vi "plot_read_output_file.vi"(9 "TMP Filepath":path, 10 "Plot Tree":refnum<vi>, 11 "Output File Loaded?":refnum<vi>) -> (3 "# Lines Plot":i32)   [LabVIEW 2019]
uses:
  lib/libOutputReader.so
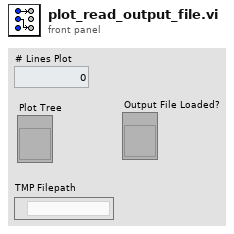
[diagram p1: front panel]
types:
  T1 = cluster{string, string[], "Child Tag":string, i32, "Child Only?":bool, i32}
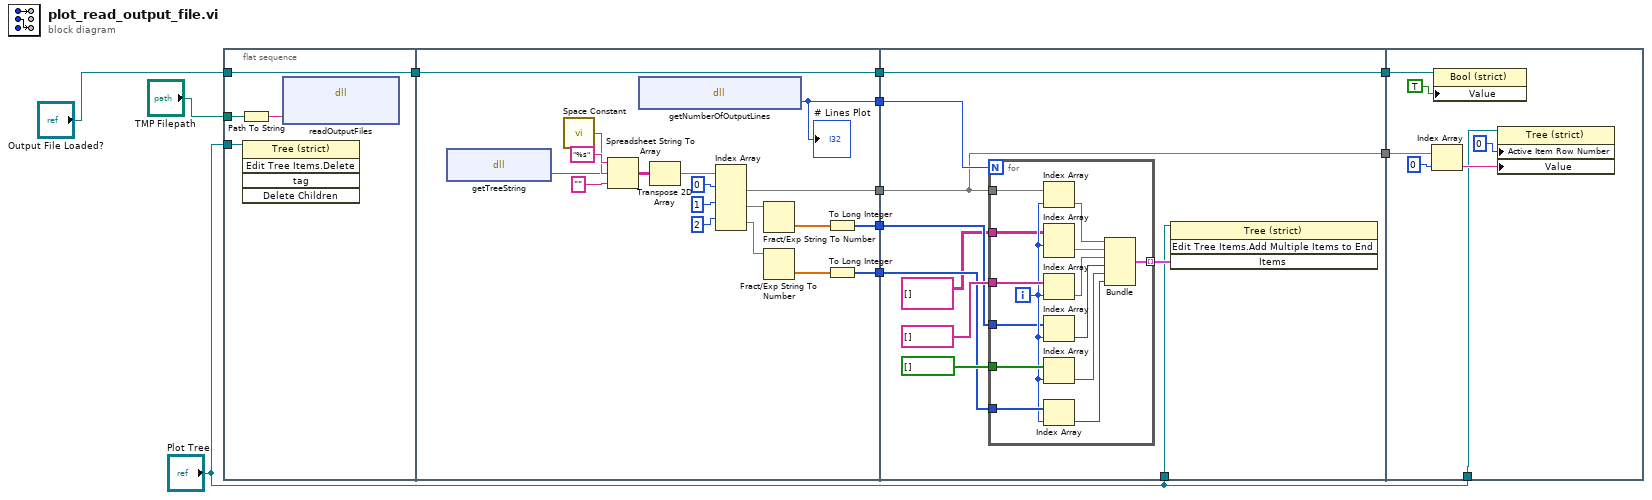
[diagram p0: block diagram]
diagram:
  n1 = flat-sequence {
    tunnel: "Plot Tree" -> [w15]
    tunnel: "TMP Filepath" -> [w14]
    tunnel: [w12] -> w4
    tunnel: "Output File Loaded?" -> [w12]
    tunnel: [w24] -> w11
    tunnel: [w22] -> w10
    tunnel: [w20] -> w9
    tunnel: [w33] -> w8
    tunnel: w4 -> [w32]
    tunnel: [w32] -> w3
    tunnel: w11 -> [w37]
    tunnel: w10 -> [w40]
    tunnel: w9 -> [w39]
    tunnel: w8 -> [w38]
    tunnel: [w37] -> w7
    tunnel: "Plot Tree" -> [w36]
    tunnel: w3 -> [w34]
    tunnel: [w34] -> w2
    tunnel: w7 -> [w62]
    tunnel: "Plot Tree" -> [w60]
    tunnel: w2 -> [w58]
    frame #0 {
      n2 = Path To String(path=w14) -> (string=w13:string)
      n3 = invoke on="Invoke Node" class="Tree (strict)" method="Edit Tree Items.Delete"(reference=w15) -> ()  [unwired: 4 in, 5 out]
      n4 = dll-call lib="home/paul/Schreibtisch/Biogas_plant_setup/lib/libOutputReader.so" fn="readOutputFiles"("tmp_filepath"=w13) -> ()  [unwired: 5 in, 2 out]
    }
    frame #1 {
      n5 = dll-call lib="home/paul/Schreibtisch/Biogas_plant_setup/lib/libOutputReader.so" fn="getTreeString"() -> ("plotTreeString"=w25:string)  [unwired: 3 in, 2 out]
      n6 = call <vilib>:"Space Constant.vi"() -> ("String"=w28:string)
      n7 = Spreadsheet String To Array(delimiter (Tab)=w28, format string="%s", spreadsheet string=w25, array type (2D Dbl)="") -> (array=w29:string[][])
      n8 = dll-call lib="home/paul/Schreibtisch/Biogas_plant_setup/lib/libOutputReader.so" fn="getNumberOfOutputLines"() -> ("numLines"=w33:i32)  [unwired: 3 in, 2 out]
      "# Lines Plot" <- w33
      n9 = Transpose 2D Array(2D array=w29) -> (transposed array=w26:string[][])
      n10 = Index Array(array=w26, index (row) #1=0 ("index (row)"), index (row) #2=1 ("index (row)"), index (row) #3=2 ("index (row)")) -> (element #1=w24:string[], element #2=w18:string[], element #3=w16:string[])  [unwired: 3 in]
      n11 = Fract/Exp String To Number(string=w18) -> (number=w23:dbl[])  [unwired: 3 in, 1 out]
      n12 = Fract/Exp String To Number(string=w16) -> (number=w21:dbl[])  [unwired: 3 in, 1 out]
      n13 = To Long Integer(number=w23) -> (32bit integer=w22:i32[])
      n14 = To Long Integer(number=w21) -> (32bit integer=w20:i32[])
    }
    frame #2 {
      n15 = for {
        N: w38 -> [_]
        tunnel: w37 -> [w57]
        tunnel: string[] [] ("Child Tag") -> [w56]
        tunnel: w40 -> [w44]
        tunnel: bool[] [] ("Child Only?") -> [w55]
        tunnel: w39 -> [w54]
        tunnel: [w48] -> w43 mode=indexing
        tunnel: string[][] [] -> [w46]
        i -> [w47]
        n16 = Index Array(array=w57, index=w47) -> (element=w53:string)
        n17 = Index Array(array=w46, index (row)=w47) -> (element=w45:string[])  [unwired: 1 in]
        n18 = Index Array(array=w56, index=w47) -> (element=w52:string)
        n19 = Index Array(array=w44, index=w47) -> (element=w51:i32)
        n20 = Index Array(array=w55, index=w47) -> (element=w50:bool)
        n21 = Index Array(array=w54, index=w47) -> (element=w49:i32)
        n22 = Bundle(w53, w45, "Child Tag"=w52, w51, "Child Only?"=w50, w49) -> (w48:T1)  [unwired: 1 in]
      }
      n23 = invoke on="Invoke Node" class="Tree (strict)" method="Edit Tree Items.Add Multiple Items to End"(reference=w36, "Items"=w43) -> ()  [unwired: 2 in, 4 out]
    }
    frame #3 {
      n24 = Index Array(array=w62, index=0) -> (element=w61:string)
      n25 = property class="Bool (strict)"(reference=w58, "Value"=TRUE) -> ()  [unwired: 1 in, 2 out]
      n26 = property on="Property Node" class="Tree (strict)"(reference=w60, "Active Item Row Number"=0 ("Active Item:Row Number"), "Value"=w61) -> ()  [unwired: 1 in, 2 out]
    }
  }
